vi "Read.vi"(8 "error in (no error)":errorcluster, 11 "Simulated Videocamera in":refnum<class "Simulated Videocamera.lvclass">) -> (0 "error out":errorcluster, 1 "timed out?":bool, 2 "Data":refnum<class "AbstractData.lvclass">, 3 "Simulated Videocamera out":refnum<class "Simulated Videocamera.lvclass">)   [LabVIEW 2014, in "Simulated Videocamera.lvclass"]
uses:
  Simulated Videocamera.lvclass
  Framework/Model/Data/AbstractData/AbstractData.lvclass
  Simulated Videocamera.lvclass/Simulated Videocamera.ctl
  Framework/Interfaces/Observable Actor/Observable Actor.lvclass
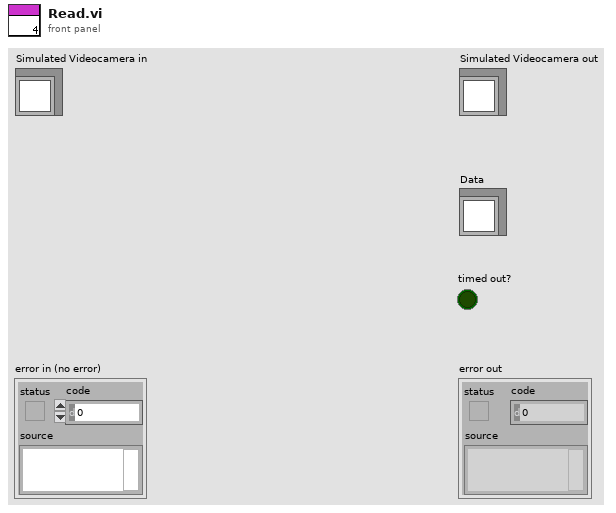
[diagram p1: front panel]
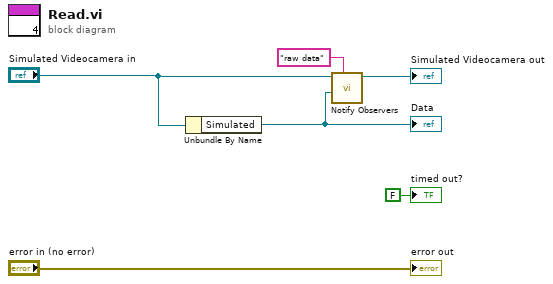
[diagram p0: block diagram]
diagram:
  n1 = Unbundle By Name("Simulated Videocamera in") -> ("Simulated"=w1:refnum<class "Data2D.lvclass">)
  "Data" <- w1
  n2 = call "Notify Observers.vi"("name"="raw data", "value"=w1, "Observable Actor in"="Simulated Videocamera in") -> ("Observable Actor out"=→"Simulated Videocamera out":refnum<class "Simulated Videocamera.lvclass">)  [unwired: 7 in, 1 out]
  "error out" <- "error in (no error)"
  "timed out?" <- FALSE ("timed out?")
